vi "Get Subscribers.vi"(8 "error in (no error)":errorcluster, 10 "Topic":string, 11 "Measure Object in":refnum<class "Measure Object.lvclass">) -> (0 "error out":errorcluster, 2 "Subscribers":refnum<class "Message Enqueuer.lvclass">[](array[class]), 3 "Measure Object out":refnum<class "Measure Object.lvclass">)   [LabVIEW 2015, in "Measure Object.lvclass"]
uses:
  Measure Object.lvclass
  <vilib>/ActorFramework/Message Enqueuer/Message Enqueuer.lvclass
  Measure Object.lvclass/Measure Object.ctl
  BroadcastBroker/BroadcastBroker.lvclass
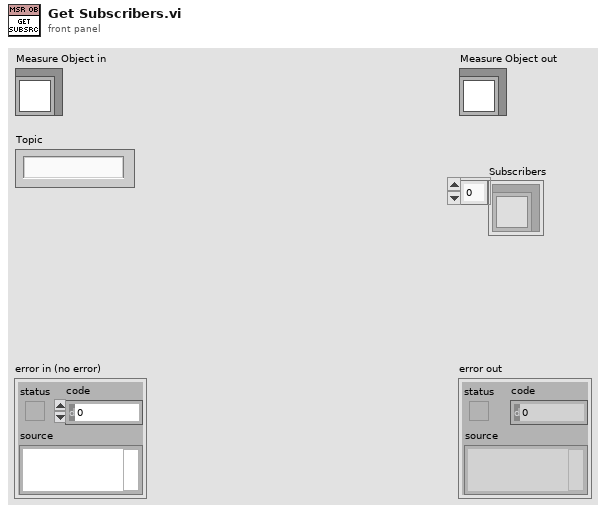
[diagram p1: front panel]
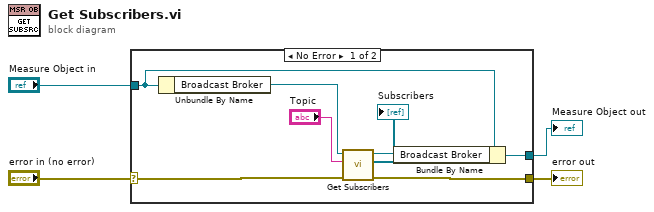
[diagram p0: block diagram]
diagram:
  n1 = case shown="No Error" "error in (no error)" {
    selector: "error in (no error)" -> [w9 w14]
    tunnel: [w8 w14] -> w3
    tunnel: [w7 w13] -> w1
    tunnel: "Measure Object in" -> [w12 w13]
    frame No Error {
      n2 = Unbundle By Name(w12) -> ("Broadcast Broker"=w11:refnum<class "BroadcastBroker.lvclass">)
      n3 = call-dynamic "Get Subscribers.vi"("error in (no error)"=w9, "Topic"="Topic", "Broadcaster in"=w11) -> ("error out"=w8:errorcluster, "Subscribers"=→"Subscribers":refnum<class "Message Enqueuer.lvclass">[], "Broadcaster out"=w6:refnum<class "BroadcastBroker.lvclass">)  [unwired: 5 in, 1 out]
      n4 = Bundle By Name(cluster=w12, "Broadcast Broker"=w6) -> (w7:refnum<class "Measure Object.lvclass">)
    }
    frame Error {
    }
  }
  "error out" <- w3
  "Measure Object out" <- w1
